vi "chart axis set reverse.vi"(8 "error in (no error)":errorcluster, 11 "axis":u32) -> (0 "error out":errorcluster)   [LabVIEW 2015, in "xlsxwriter.lvlib"]
doc: "void chart_axis_set_reverse(lxw_chart_axis axis);"
uses:
  xlsxwriter.lvlib
  xlsxwriter.dll
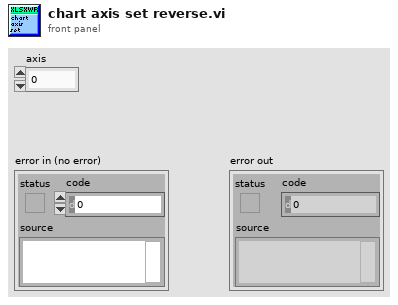
[diagram p1: front panel]
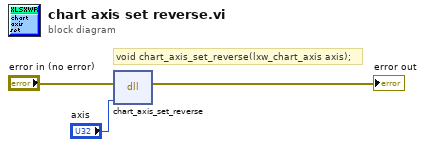
[diagram p0: block diagram]
diagram:
  # "void chart_axis_set_reverse(lxw_chart_axis axis);"
  n1 = dll-call lib="C:/Users/WDAGUtilityAccount/Desktop/lv_vis_added_cell/xlsxwriter.*" fn="chart_axis_set_reverse"(error in="error in (no error)", "axis"="axis") -> (error out=→"error out":errorcluster)  [unwired: 4 in, 1 out]
